vi "LIDAR V2 FPGA Main.vi"() -> ()   [LabVIEW 2013]
uses:
  <vilib>/Platform/TimedLoop/XDataNode/XDataNode.xnode
  <vilib>/Platform/TimedLoop/XDataNode/nitl_modes.ctl
  <vilib>/Platform/TimedLoop/XDataNode/XDNodeRunTimeDep.lvlib
  <vilib>/Platform/TimedLoop/XDataNode/wakeup.ctl
  <vilib>/Platform/TimedLoop/XDataNode/timing_clust.ctl
  <vilib>/eio/EIONode/EIONode.xnode
  <vilib>/rvi/eio/common/nirviEmuTemplateMethod_errors.vi
  <vilib>/rvi/DataTransferAndStorage/Container/XNode/niFpgaContainer.xnode
  <vilib>/rvi/FIFO/Fifo_Resource/nirvififoEmulationWrite.vi
  Controls/FPGA Nain State.ctl
  LIDAR V2 Globals.vi
  Controls/Add&Data&Ai Typedef.ctl
  Controls/Add&Data Typedef.ctl
  <vilib>/rvi/FIFO/Fifo_Resource/nirvififoEmulationRead.vi
  Controls/Scan Format Typedaf.ctl
panel:
  out "SimOut":i16
  in  "PulseUpClck":u16=20
  in  "PulseWaitClck":u16=40
  in  "GenPulse":bool
  out "SPI Idle":bool
  out "PLL Locked":bool
  in  "Clock":u8=1
  out "PLL Counter":i32
  in  "IO Module\\Apply Settings":bool
  out "InitMem":bool
  out "PulseIndex":i16
  in  "NextLedEn":bool
  in  "SingleCycle":bool
  out "PulseEnd":bool
  out "LedAddress":u16
  in  "ScanFormat":T1=enum."FullScanPerLed"
  in  "SamplingEnable":bool
  out "MainState":T2
  in  "PulsePerLed":i16=10
  out "IterReset":u16 format="%.0b"
  in  "SampPerPulse":i16=100
  in  "ActiveLedIndex":u16
  out "10thIndex":u8
  in  "MemSel":bool
  in  "EnAI":bool
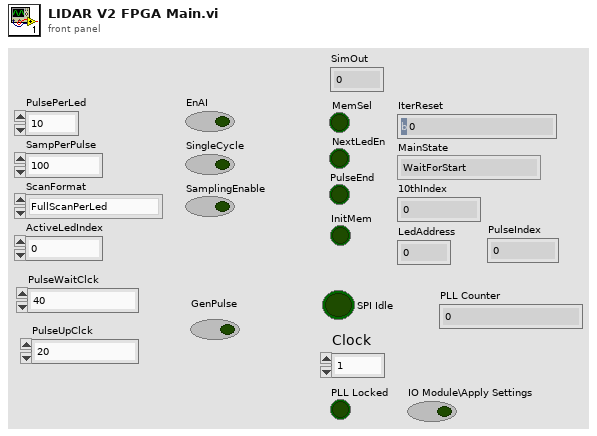
[diagram p1: front panel]
types:
  T1 = typedef "Scan Format Typedaf.ctl" = enum16{"1PulsePerLed", "FullScanPerLed"}
  T2 = typedef "FPGA Nain State.ctl" = enum16{"WaitForStart", "SetProcParams", "SelectActiveLed", "ActivatePulse", "WaitForPulseEnd", "WaitForAlgoStart", "SingleCycleEnd"}
  T3 = typedef "XDNodeRunTimeDep.lvlib/timing_clust.ctl" = cluster{"Expected End [f-1]":u64, "Actual End [f-1]":u64, "Finished Late? [f-1]":bool, "Expected End [i-1]":u64, "Actual End [i-1]":u64, "Finished Late? [i-1]":bool, "Expected Start [i]":u64, "Actual Start [i]":u64, "Expected Start [f]":u64, "Actual Start [f]":u64, "Source Name":string, "Structure Name":string, "Period":i64, "Deadline":i64, "Offset":i64, "Start":i64, "Priority":i32, "Timeout":i32, "Mode":T4, "Wakeup Reason":T5, "Error":errorcluster, "Source Type":string, "Secondary Source Type":string, "Global End Time":u64, "Global Start Time":u64, "Frame Duration":u64, "Iteration Duration":u64, "Assigned CPU":i32, "I/O Scan Engine Mode":u32}
  T4 = typedef "XDNodeRunTimeDep.lvlib/nitl_modes.ctl" = enum32{"No Change", "Process missed periods, maintain original phase", "Discard missed periods, maintain original phase", "Process missed periods, ignore original phase", "Discard missed periods, ignore original phase"}
  T5 = typedef "XDNodeRunTimeDep.lvlib/wakeup.ctl" = enum32{"Normal", "Aborted", "Asynchronous wakeup", "Timing source error", "Timed loop error", "Timeout"}
  T6 = typedef "Add&Data Typedef.ctl" = cluster{"Add":i16, "Data":fxp<+/-,22,22>}
  T7 = typedef "Add&Data&Ai Typedef.ctl" = cluster{"Add":i16, "Ai":fxp<+/-,16,16>, "Init":bool}
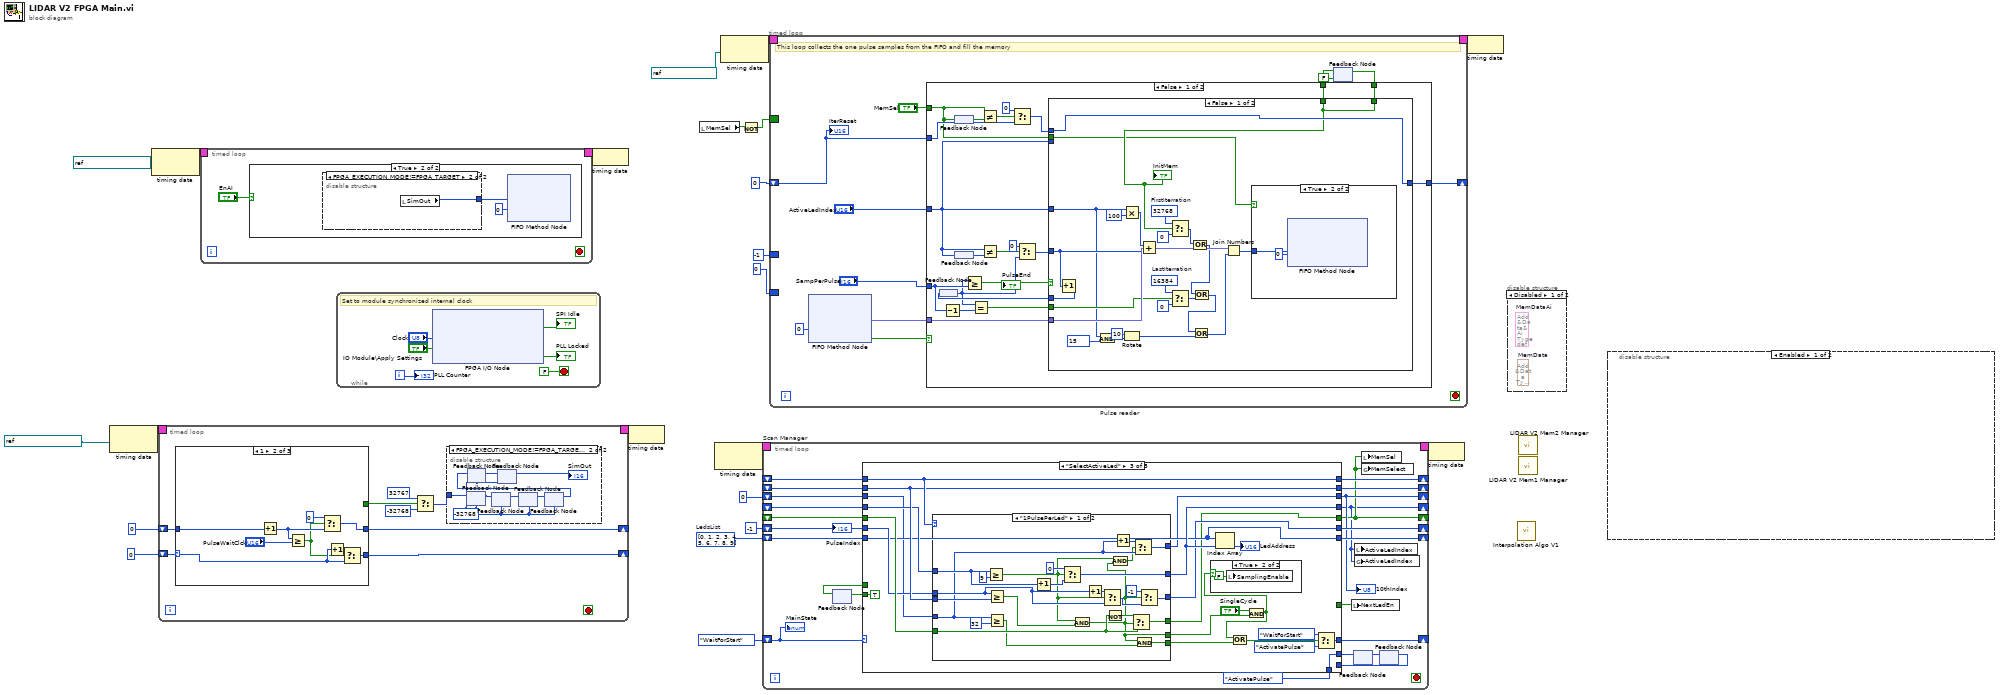
[diagram p0: block diagram]
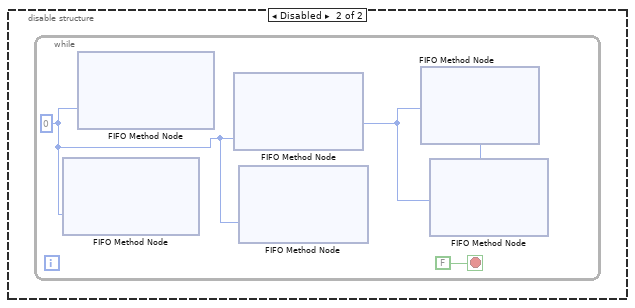
[diagram p2: hidden frame]
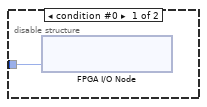
[diagram p3: hidden frame]
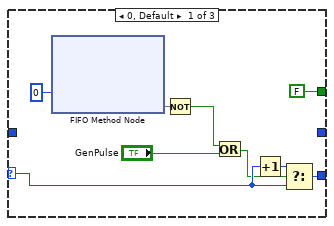
[diagram p4: hidden frame]
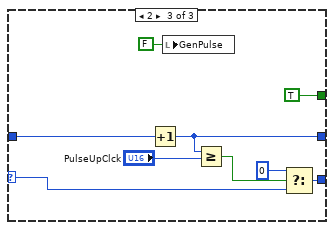
[diagram p5: hidden frame]
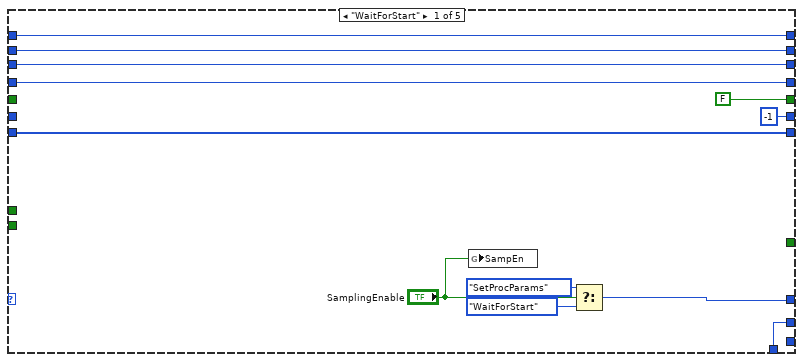
[diagram p7: hidden frame]
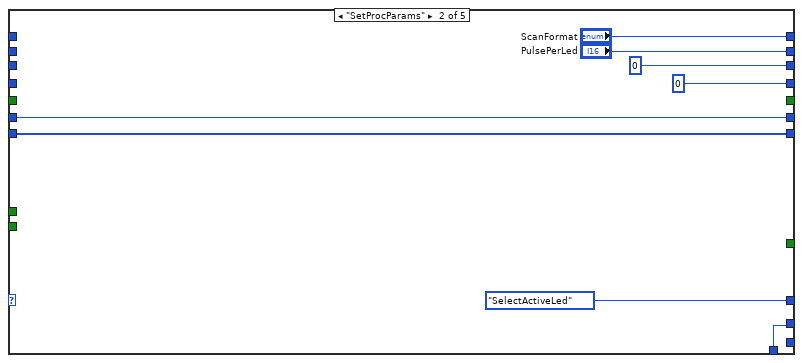
[diagram p8: hidden frame]
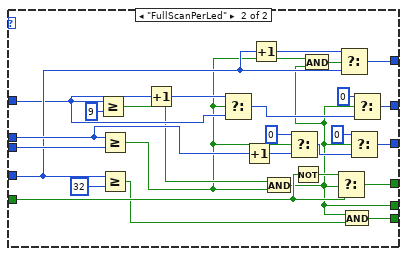
[diagram p10: hidden frame]
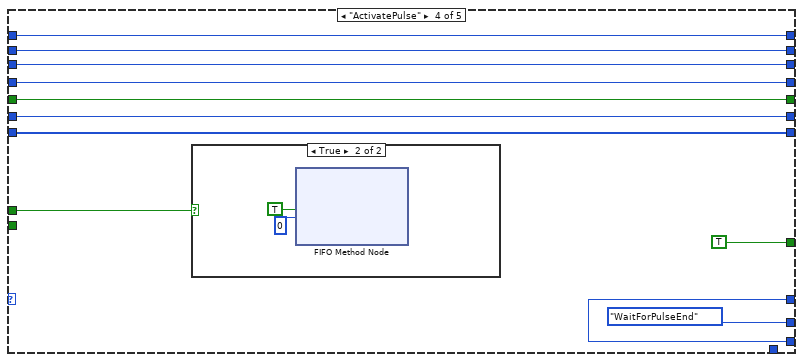
[diagram p11: hidden frame]
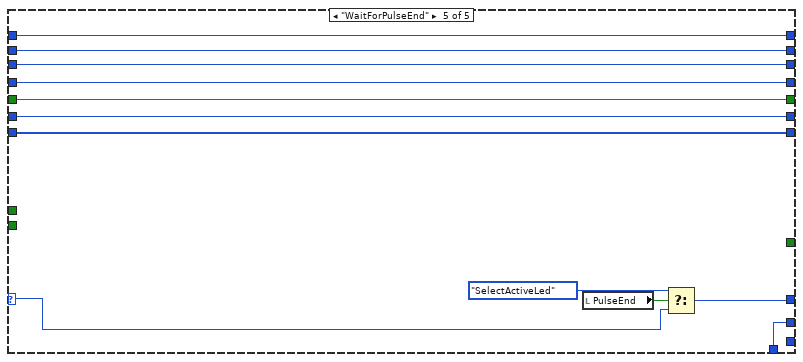
[diagram p13: hidden frame]
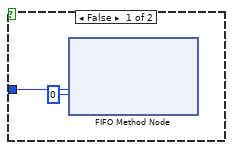
[diagram p14: hidden frame]
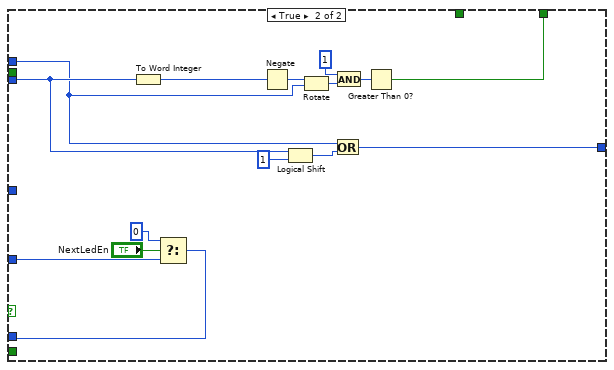
[diagram p15: hidden frame]
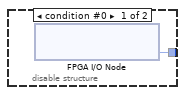
[diagram p18: hidden frame]
diagram:
  w7 = u16[] [0, 1, 2, 3, 4, 5, 6, 7, 8, 9]  # LedsList
  n1 = node-c288(refnum<k21> "IO Module Clock 0" ("Source Name")) -> (w5:T3)
  n2 = node-c288(refnum<k21> "IO Module Clock 0" ("Source Name")) -> (w22:T3)
  n3 = timed-loop {
    timing: w5 -> [_]
    timing-out: [_] -> w4
    shift-right: [w29] -> _
    shift-left: i16 0 -> [w30]
    shift-right: [w27] -> _
    shift-left: u16 0 -> [w28]
    stop <- _ stop-if-true
    n4 = case shown="1" w30 {
      selector: w30 -> [w46 w54 w61]
      tunnel: [w47 w55 w62] -> w29
      tunnel: w28 -> [_ w57 w66]
      tunnel: [_ w51 w65] -> w27
      tunnel: [FALSE _ TRUE] -> w24
      frame 0, Default {
        n5 = xnode ("FIFO Method Node")("Timeout"=0) -> ("Timed Out?"=w42)  [unwired: 1 in, 2 out]
        n6 = Not(x=w42) -> (.not. x?=w41:bool)
        n7 = Or(x=w41, y="GenPulse") -> (x .or. y?=w43:bool)
        n8 = Increment(x=w46) -> (x+1=w45:i16)
        n9 = Select(t=w45, s=w43, f=w46) -> (s? t:f=w47:i16)
      }
      frame 1 {
        n10 = Increment(x=w57) -> (x+1=w52:u16)
        n11 = Greater Or Equal?(x=w52, y="PulseWaitClck") -> (x >= y?=w50:bool)
        n12 = Select(t=u16 0, s=w50, f=w52) -> (s? t:f=w51:u16)
        n13 = Increment(x=w54) -> (x+1=w53:i16)
        n14 = Select(t=w53, s=w50, f=w54) -> (s? t:f=w55:i16)
      }
      frame 2 {
        n15 = Increment(x=w66) -> (x+1=w65:u16)
        n16 = local write "GenPulse"(FALSE ("GenPulse")) -> ()
        n17 = Greater Or Equal?(x=w65, y="PulseUpClck") -> (x >= y?=w63:bool)
        n18 = Select(t=i16 0, s=w63, f=w61) -> (s? t:f=w62:i16)
      }
    }
    n19 = Select(t=i16 32767 ("IO Module\\AO 0"), s=w24, f=i16 -32768 ("IO Module\\AO 0")) -> (s? t:f=w23:i16)
    n20 = disable-structure shown="FPGA_EXECUTION_MODE!=FPGA_TARGET" {
      disable-tunnel: w23 -> [w31 w39]
      frame condition #0 {
        n21 = xnode "FPGA I/O Node"("IO Module\\AO 0"=w31) -> ()  [unwired: 1 in, 1 out]
      }
      frame condition #1 (active) {
        w33 = i16 -32768 ("IO Module\\AO 0")
        n22 = feedback-in #1(w39) -> ()
        n23 = feedback #1(w33) -> (w38:i16)
        n24 = feedback #2(w33) -> (w34:i16)
        n25 = feedback #3(w33) -> (w37:i16)
        n26 = feedback-in #3(w38) -> ()
        n27 = feedback #4(w33) -> (→"SimOut":i16)
        n28 = feedback-in #4(w34) -> ()
        n29 = feedback #5(w33) -> (w36:i16)
        n30 = feedback-in #5(w37) -> ()
        n31 = feedback #6(w33) -> (w35:i16)
        n32 = feedback-in #2(w35) -> ()
        n33 = feedback-in #6(w36) -> ()
      }
    }
  }
  n34 = timed-loop {
    timing: w22 -> [_]
    timing-out: [_] -> w21
    stop <- _ stop-if-true
    n35 = case shown="True" "EnAI" {
      frame False {
      }
      frame True {
        n36 = disable-structure shown="FPGA_EXECUTION_MODE!=FPGA_TARGET" {
          disable-tunnel: [w72 w73] -> w70
          frame condition #0 {
            n37 = xnode "FPGA I/O Node"() -> ("IO Module\\AI 0"=w72:i16)  [unwired: 1 in, 1 out]
          }
          frame condition #1 (active) {
            n38 = local read "SimOut"() -> (w73:i16)
          }
        }
        n39 = xnode ("FIFO Method Node")("Element"=w70, "Timeout"=0) -> ()  [unwired: 1 in, 2 out]
      }
    }
  }
  n40 = while {
    i -> [w78]
    stop <- FALSE stop-if-true
    # "Set to module synchronized internal clock"
    n41 = xnode "FPGA I/O Node"("IO Module\\Clock Select"="Clock", "IO Module\\Apply Settings"="IO Module\\Apply Settings") -> ("IO Module\\SPI Idle"=→"SPI Idle":bool, "IO Module\\PLL Locked"=→"PLL Locked":bool)  [unwired: 4 in, 4 out]
    "PLL Counter" <- w78
  }
  n42 = node-c288(w21) -> ()
  n43 = node-c288(w4) -> ()
  n44 = local read "MemSel"() -> (w14:bool)
  n45 = node-c288() -> (w11:T3)  [unwired: 1 in]
  n46 = node-c288(refnum<k21> "100 MHz Clock" ("Source Name")) -> (w19:T3)
  n47 = Not(x=w14) -> (.not. x?=w13:bool)
  n48 = timed-loop "Scan Manager" {
    timing: w11 -> [_]
    timing-out: [_] -> w10
    shift-right: [w103] -> _
    shift-left: FPGA_Nain_State."WaitForStart" ("MainState") -> [w104]
    shift-right: [w102] -> _
    shift-left: _ -> [w100]
    shift-right: [w101] -> _
    shift-left: _ -> [w99]
    shift-right: [w92] -> _
    shift-left: u8 0 ("10thIndex") -> [w98]
    shift-right: [w82] -> _
    shift-left: _ -> [w97]
    shift-right: [w86] -> _
    shift-left: _ -> [w96]
    shift-right: [w95] -> _
    shift-left: i16 -1 -> [w85]
    shift-right: [w93] -> _
    shift-left: w7 -> [w94]
    stop <- _ stop-if-true
    n49 = feedback #7() -> (w83:bool)  [unwired: 1 in]
    n50 = feedback #8() -> (w89:T2)  [unwired: 1 in]
    n51 = feedback #9() -> (w88:T2)  [unwired: 1 in]
    n52 = case shown="\"SelectActiveLed\"" w104 {
      selector: w104 -> [_ _ _ _ w216]
      tunnel: [w114 FPGA_Nain_State."SelectActiveLed" ("MainState") w130 w199 w215] -> w103
      tunnel: [w113 "ScanFormat" w146 w208 w222] -> w102
      tunnel: [w112 "PulsePerLed" w144 w207 w221] -> w101
      tunnel: w100 -> [w113 _ w146 w208 w222]
      tunnel: w99 -> [w112 _ w144 w207 w221]
      tunnel: [w111 u8 0 ("10thIndex") w133 w206 w220] -> w92
      tunnel: w98 -> [w111 _ w134 w206 w220]
      tunnel: [w110 u16 0 ("ActiveLedIndex") w141 w205 w219] -> w82
      tunnel: w97 -> [w110 _ w142 w205 w219]
      tunnel: [FALSE _ w137 w204 w218] -> w86
      tunnel: w96 -> [_ _ w145 w204 w218]
      tunnel: [i16 -1 ("t") w119 w138 w203 w213] -> w95
      tunnel: w85 -> [_ w119 w143 w203 w213]
      tunnel: w94 -> [w108 w118 w140 w202 w212]
      tunnel: [w108 w118 w140 w202 w212] -> w93
      tunnel: [_ _ _ TRUE ("SampEnable") _] -> w91
      tunnel: [w107 w117 w132 FPGA_Nain_State."WaitForPulseEnd" ("MainState") w211] -> w90
      tunnel: w88 -> [_ _ _ w199 _]
      tunnel: FPGA_Nain_State."ActivatePulse" ("MainState") -> [w107 w117 w132 _ w211]
      tunnel: [_ _ TRUE _ _] -> w84
      tunnel: w83 -> [_ _ _ w198 _]
      frame "WaitForStart" {
        n53 = global write "LIDAR V2 Globals.vi" "SampEn"("SamplingEnable") -> ()
        n54 = Select(t=FPGA_Nain_State."SetProcParams" ("MainState"), s="SamplingEnable", f=FPGA_Nain_State."WaitForStart" ("MainState")) -> (s? t:f=w114:T2)
      }
      frame "SetProcParams" {
      }
      frame "SelectActiveLed" {
        n55 = case shown="\"1PulsePerLed\"" w146 {
          tunnel: w145 -> [w163 w193]
          tunnel: w134 -> [w156 w188]
          tunnel: w144 -> [w166 w195]
          tunnel: w142 -> [w169 w179]
          tunnel: w143 -> [w165 w194]
          tunnel: [w157 w175] -> w141
          tunnel: [w152 w177] -> w138
          tunnel: [w160 w191] -> w137
          tunnel: [w158 w189] -> w128
          tunnel: [w154 w186] -> w133
          tunnel: [w148 w172] -> w131
          frame "1PulsePerLed" {
            n56 = Greater Or Equal?(x=w169, y=u16 9) -> (x >= y?=w150:bool)
            n57 = Greater Or Equal?(x=w165, y=w166) -> (x >= y?=w161:bool)
            n58 = Greater Or Equal?(x=w156, y=u8 32) -> (x >= y?=w159:bool)
            n59 = Increment(x=w169) -> (x+1=w168:u16)
            n60 = Select(t=u16 0, s=w150, f=w168) -> (s? t:f=w157:u16)
            n61 = And(x=w150, y=w161) -> (x .and. y?=w148:bool)
            n62 = Increment(x=w165) -> (x+1=w164:i16)
            n63 = Select(t=w164, s=w150, f=w165) -> (s? t:f=w153:i16)
            n64 = Not(x=w163) -> (.not. x?=w162:bool)
            n65 = And(x=w150, y=w148) -> (x .and. y?=w149:bool)
            n66 = Increment(x=w156) -> (x+1=w155:u8)
            n67 = Select(t=w162, s=w148, f=w163) -> (s? t:f=w160:bool)
            n68 = Select(t=w155, s=w149, f=w156) -> (s? t:f=w154:u8)
            n69 = And(x=w148, y=w159) -> (x .and. y?=w158:bool)
            n70 = Select(t=i16 -1, s=w148, f=w153) -> (s? t:f=w152:i16)
          }
          frame "FullScanPerLed" {
            n71 = Greater Or Equal?(x=w179, y=u16 9) -> (x >= y?=w178:bool)
            n72 = Greater Or Equal?(x=w194, y=w195) -> (x >= y?=w173:bool)
            n73 = Greater Or Equal?(x=w188, y=u8 32) -> (x >= y?=w190:bool)
            n74 = Increment(x=w179) -> (x+1=w180:u16)
            n75 = Select(t=w180, s=w173, f=w179) -> (s? t:f=w176:u16)
            n76 = Increment(x=w194) -> (x+1=w182:i16)
            n77 = Increment(x=w188) -> (x+1=w187:u8)
            n78 = And(x=w178, y=w173) -> (x .and. y?=w172:bool)
            n79 = Select(t=i16 0, s=w173, f=w182) -> (s? t:f=w185:i16)
            n80 = Not(x=w193) -> (.not. x?=w192:bool)
            n81 = And(x=w173, y=w172) -> (x .and. y?=w183:bool)
            n82 = Select(t=w192, s=w172, f=w193) -> (s? t:f=w191:bool)
            n83 = Select(t=w187, s=w183, f=w188) -> (s? t:f=w186:u8)
            n84 = And(x=w172, y=w190) -> (x .and. y?=w189:bool)
            n85 = Select(t=i16 0, s=w172, f=w185) -> (s? t:f=w177:i16)
            n86 = Select(t=u16 0, s=w172, f=w176) -> (s? t:f=w175:u16)
          }
        }
        n87 = Index Array(array=w140, index=w141) -> (element=→"LedAddress":u16)
        n88 = And(x="SingleCycle", y=w131) -> (x .and. y?=w127:bool)
        n89 = case shown="True" w127 {
          frame False {
          }
          frame True {
            n90 = local write "SamplingEnable"(FALSE ("SamplingEnable")) -> ()
          }
        }
        n91 = Or(x=w127, y=w128) -> (x .or. y?=w126:bool)
        n92 = Select(t=FPGA_Nain_State."WaitForStart" ("MainState"), s=w126, f=FPGA_Nain_State."ActivatePulse" ("MainState")) -> (s? t:f=w130:T2)
      }
      frame "ActivatePulse" {
        n93 = case shown="True" w198 {
          frame False {
          }
          frame True {
            n94 = xnode ("FIFO Method Node")("Element"=TRUE ("GenPulse"), "Timeout"=0) -> ()  [unwired: 1 in, 2 out]
          }
        }
      }
      frame "WaitForPulseEnd" {
        n95 = local read "PulseEnd"() -> (w217:bool)
        n96 = Select(t=FPGA_Nain_State."SelectActiveLed", s=w217, f=w216) -> (s? t:f=w215:T2)
      }
    }
    "10thIndex" <- w92
    n97 = feedback-in #7(w84) -> ()
    n98 = local write "NextLedEn"(w91) -> ()
    n99 = feedback-in #8(w90) -> ()
    n100 = local write "ActiveLedIndex"(w82) -> ()
    n101 = global write "LIDAR V2 Globals.vi" "ActiveLedIndex"(w82) -> ()
    n102 = local write "MemSel"(w86) -> ()
    n103 = global write "LIDAR V2 Globals.vi" "MemSelect"(w86) -> ()
    n104 = feedback-in #9(w89) -> ()
    "MainState" <- w104
    "PulseIndex" <- w85
  }
  n105 = timed-loop "Pulse reader" {
    timing: w19 -> [_]
    timing-out: [_] -> w18
    border: i16 -1 ("#Cycle") -> [_]
    border: u16 0 -> [_]
    shift-right: [w231] -> _
    shift-left: u16 0 -> [w229]
    border: w13 -> [_]
    stop <- _ stop-if-true
    # "This loop collects the one pulse samples from the FIFO and fill the memory"
    n106 = xnode ("FIFO Method Node")("Timeout"=0) -> ("Element"=w234:fxp<+/-,16,16>, "Timed Out?"=w233:bool)  [unwired: 1 in, 1 out]
    n107 = feedback #10(FALSE) -> (w227:bool)
    n108 = case shown="False" w233 {
      tunnel: w234 -> [w241 _]
      tunnel: "ActiveLedIndex" -> [w245 _]
      tunnel: "SampPerPulse" -> [w240 _]
      tunnel: [w253 w302] -> w231
      tunnel: w229 -> [w249 w302]
      tunnel: [w243 w301] -> w228
      tunnel: w227 -> [w242 w301]
      tunnel: "MemSel" -> [w236 _]
      frame False {
        n109 = feedback #11() -> (w239:u16)
        n110 = Decrement(x=w240) -> (x-1=w238:i16)
        n111 = feedback #12() -> (w251:bool)
        n112 = feedback-in #12(w236) -> ()
        n113 = feedback #13() -> (w256:u16)
        n114 = feedback-in #13(w245) -> ()
        n115 = Greater Or Equal?(x=w239, y=w240) -> (x >= y?=w248:bool)
        "PulseEnd" <- w248
        n116 = Equal?(x=w239, y=w238) -> (x = y?=w237:bool)
        n117 = Not Equal?(x=w245, y=w256) -> (x != y?=w246:bool)
        n118 = Not Equal?(x=w236, y=w251) -> (x != y?=w252:bool)
        n119 = Select(t=u16 0, s=w252, f=w249) -> (s? t:f=w244:u16)
        n120 = Select(t=u16 0, s=w246, f=w239) -> (s? t:f=w247:u16)
        n121 = case shown="False" w248 {
          tunnel: w241 -> [w280 _]
          tunnel: [w281 w299] -> w254
          tunnel: [w275 w300] -> w253
          tunnel: w244 -> [w275 w288]
          tunnel: w245 -> [_ w289]
          tunnel: w247 -> [w277 w298]
          tunnel: w245 -> [w264 _]
          tunnel: [w274 w287] -> w243
          tunnel: w242 -> [w274 _]
          tunnel: w237 -> [w267 _]
          tunnel: w236 -> [w257 _]
          frame False {
            w268 = u16 16384  # LastIterration
            w272 = u16 32768  # FirstIterration
            n122 = Increment(x=w277) -> (x+1=w281:u16)
            n123 = And(x=w264, y=u16 15) -> (x .and. y?=w262:u16)
            n124 = Rotate(1:w262, 2:i16 10 ("y")) -> (0:w260:u16)
            n125 = Multiply(x=w264, y=u16 100) -> (x*y=w278:u16)
            n126 = Add(x=w278, y=w277) -> (x+y=w276:u16)
            n127 = Select(t=w272, s=w274, f=u16 0 ("x")) -> (s? t:f=w273:u16)
            n128 = Select(t=w268, s=w267, f=u16 0 ("x")) -> (s? t:f=w266:u16)
            n129 = Or(x=w273, y=w276) -> (x .or. y?=w265:u16)
            n130 = Or(x=w265, y=w266) -> (x .or. y?=w259:u16)
            n131 = Or(x=w259, y=w260) -> (x .or. y?=w258:u16)
            n132 = Join Numbers(hi=w280, lo=w258) -> ((hi.lo)=w270:u32)
            n133 = case shown="True" w257 {
              tunnel: w270 -> [w282 w284]
              frame False {
                n134 = xnode ("FIFO Method Node")("Element"=w282, "Timeout"=0) -> ()  [unwired: 1 in, 2 out]
              }
              frame True {
                n135 = xnode ("FIFO Method Node")("Element"=w284, "Timeout"=0) -> ()  [unwired: 1 in, 2 out]
              }
            }
            "InitMem" <- w274
          }
          frame True {
            n136 = To Word Integer(number=w289) -> (16bit integer=w286:i16)
            n137 = Select(t=i16 0, s="NextLedEn", f=w298) -> (s? t:f=w299:u16)
            n138 = Negate(x=w286) -> (-x=w293:i16)
            n139 = Logical Shift(y=w289, x=u16 1) -> (x << y=w294:u16)
            n140 = Rotate(1:w288, 2:w293) -> (0:w292:u16)
            n141 = Or(x=w288, y=w294) -> (x .or. y?=w300:u16)
            n142 = And(x=u16 1, y=w292) -> (x .and. y?=w290:u16)
            n143 = Greater Than 0?(x=w290) -> (x > 0?=w287:bool)
          }
        }
        n144 = feedback-in #11(w254) -> ()
      }
      frame True {
      }
    }
    n145 = feedback-in #10(w228) -> ()
    "IterReset" <- w229
  }
  n146 = node-c288(w10) -> ()
  n147 = node-c288(w18) -> ()
  n148 = disable-structure shown="Disabled" {
    frame Disabled {
      (unwired) T6 {"Add"=0, "Data"=0.0}  # MemData
      (unwired) T7 {"Add"=0, "Ai"=0.0, "Init"=FALSE}  # MemDataAi
    }
    frame Enabled {
    }
  }
  n149 = call "Interpolation Algo V1.vi"() -> ()  [unwired: 10 in, 2 out]
  n150 = call "LIDAR V2 Mem2 Manager.vi"() -> ()  [unwired: 12 in]
  n151 = call "LIDAR V2 Mem1 Manager.vi"() -> ()  [unwired: 12 in]
  n152 = disable-structure shown="Enabled" {
    frame Enabled {
    }
    frame Disabled {
      n153 = while {
        stop <- FALSE stop-if-true
        w305 = 0 ("Timeout")
        n154 = xnode ("FIFO Method Node")("Timeout"=w305) -> ()  [unwired: 1 in, 3 out]
        n155 = xnode ("FIFO Method Node")("Timeout"=w305) -> ()  [unwired: 1 in, 3 out]
        n156 = xnode ("FIFO Method Node")("Timeout"=w305) -> ()  [unwired: 1 in, 3 out]
        n157 = xnode ("FIFO Method Node")("Timeout"=w305) -> ()  [unwired: 1 in, 3 out]
        n158 = xnode ("FIFO Method Node")("Element"=w305, "Timeout"=w305) -> ()  [unwired: 1 in, 2 out]
        n159 = xnode ("FIFO Method Node")("Element"=w305, "Timeout"=w305) -> ()  [unwired: 1 in, 2 out]
      }
    }
  }
